vi "SubSystems.vi"(8 "error in":errorcluster) -> ()   [LabVIEW 2023]
doc: "This VI calls the various robot subsystems that will then run in parallel. New subSystems will automatlically script code to make the call."
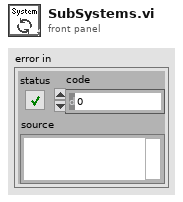
[diagram p1: front panel]
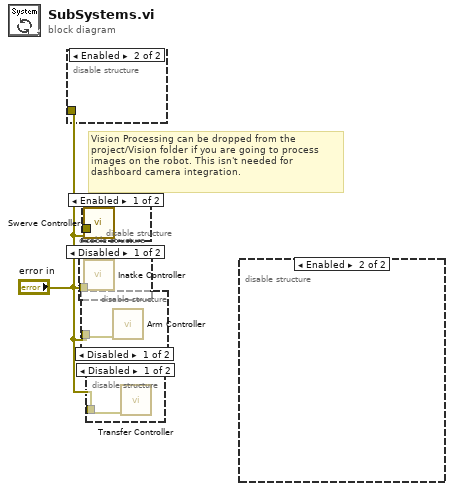
[diagram p0: block diagram]
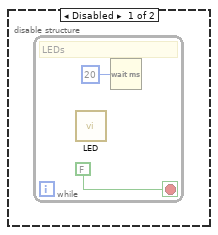
[diagram p3: hidden frame]
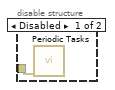
[diagram p7: hidden frame]
diagram:
  # "Vision Processing can be dropped from the\nproject/Vision folder if you are going to process\nimages on the robot. This isn't needed for\ndashboard camera integration."
  n1 = disable-structure shown="Enabled" {
    disable-tunnel: "error in" -> [w2 _]
    frame Disabled {
      n2 = call "Periodic Tasks.vi"("error in"=w2) -> ()  [unwired: 1 in, 10 out]
    }
    frame Enabled {
    }
  }
  n3 = disable-structure shown="Disabled" {
    disable-tunnel: "error in" -> [w3 _]
    frame Disabled {
      n4 = call "Inatke Controller.vi"("error in"=w3) -> ()  [unwired: 11 in]
    }
    frame Enabled {
    }
  }
  n5 = disable-structure shown="Disabled" {
    disable-tunnel: "error in" -> [w4 _]
    frame Disabled {
      n6 = call "Arm Controller.vi"("error in"=w4) -> ()  [unwired: 11 in]
    }
    frame Enabled {
    }
  }
  n7 = disable-structure shown="Enabled" {
    disable-tunnel: "error in" -> [w5 _]
    frame Enabled {
      n8 = call "Swerve Controller.vi"("error in"=w5) -> ()  [unwired: 11 in]
    }
    frame Disabled {
    }
  }
  n9 = disable-structure shown="Disabled" {
    disable-tunnel: "error in" -> [w6 _]
    frame Disabled {
      n10 = call "Transfer Controller.vi"("error in"=w6) -> ()  [unwired: 11 in]
    }
    frame Enabled {
    }
  }
  n11 = disable-structure shown="Enabled" {
    frame Disabled {
      n12 = while {
        stop <- FALSE stop-if-true
        # "LEDs"
        n13 = call "LED.vi"() -> ()  [unwired: 12 in]
        n14 = Wait (ms)(milliseconds to wait=u32 20) -> ()  [unwired: 1 out]
      }
    }
    frame Enabled {
    }
  }
